vi "Configure Spurious Emission (Limit Setup).vi"(0 "VISA resource name":refnum<visa-resource-name>, 1 "Spurious Threshold":dbl[](array[numeric]) min=-200.0 max=50.0 format="%.2f", 2 "Spurious Stop Level Mode":i32[](array[ring]) items=["Auto", "Manual"], 5 "Spurious Absolute Level Start":dbl[](array[numeric]) min=-200.0 max=50.0 format="%.2f", 7 "Spurious Absolute Level Stop":dbl[](array[numeric]) min=-200.0 max=50.0 format="%.2f", 9 "Spurious Resolution":dbl[](array[numeric]) min=0.001 max=50.0 format="%.3f", 11 "error in (no error)":errorcluster) -> (4 "VISA resource name out":refnum<visa-resource-name>, 15 "error out":errorcluster)   [LabVIEW 2020, in "Anritsu Signal Analyzer Series.lvlib"]
doc: "Configures the Limit for Spurious Emission measurement."
uses:
  Anritsu Signal Analyzer Series.lvlib
panel:
  # "dBm"
  # "dBm"
  # "dBm"
  # "dB"
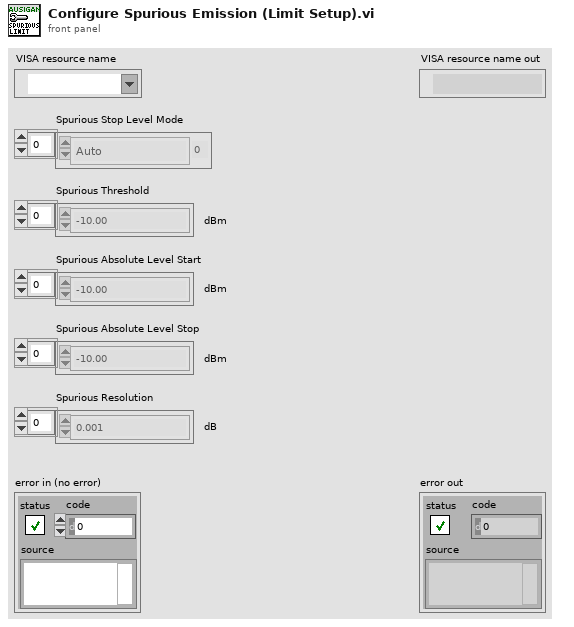
[diagram p1: front panel]
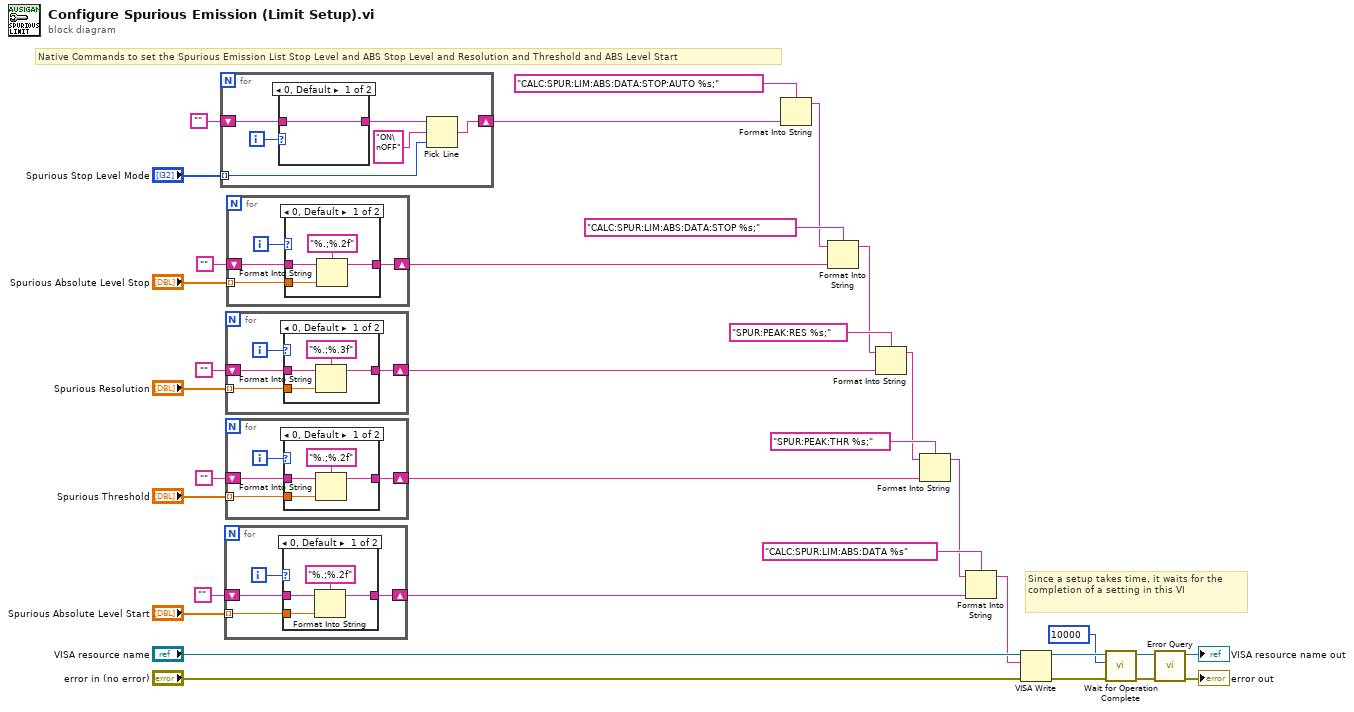
[diagram p0: block diagram]
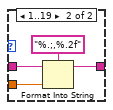
[diagram p2: hidden frame]
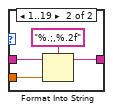
[diagram p3: hidden frame]
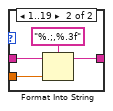
[diagram p4: hidden frame]
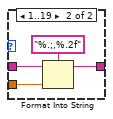
[diagram p5: hidden frame]
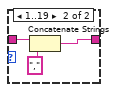
[diagram p6: hidden frame]
diagram:
  # "Since a setup takes time, it waits for the completion of a setting in this VI"
  # "Native Commands to set the Spurious Emission List Stop Level and ABS Stop Level and Resolution and Threshold and ABS Level Start"
  n1 = for {
    shift-right: [w35] -> w24
    shift-left: "" -> [w39]
    tunnel: "Spurious Stop Level Mode" -> [w36] mode=indexing
    i -> [w40]
    n2 = case shown="0, Default" w40 {
      tunnel: w39 -> [w41 w44]
      tunnel: [w41 w42] -> w37
      frame 0, Default {
      }
      frame 1..19 {
        n3 = Concatenate Strings(w44, "," ("string")) -> (w42:string)
      }
    }
    n4 = Pick Line(string ("")=w37, multi-line string="ON\nOFF" ("複数行文字列"), line index=w36) -> (output string=w35:string)
  }
  n5 = for {
    shift-right: [w45] -> w6
    shift-left: "" -> [w47]
    tunnel: "Spurious Absolute Level Start" -> [w46] mode=indexing
    i -> [w48]
    n6 = case shown="0, Default" w48 {
      tunnel: w47 -> [w51 w54]
      tunnel: [w49 w53] -> w45
      tunnel: w46 -> [w50 w55]
      frame 0, Default {
        n7 = Format Into String(format string="%.;%.2f" ("string"), initial string=w51, w50) -> (resulting string=w49:string)  [unwired: 1 in, 1 out]
      }
      frame 1..19 {
        n8 = Format Into String(format string="%.;,%.2f" ("string"), initial string=w54, w55) -> (resulting string=w53:string)  [unwired: 1 in, 1 out]
      }
    }
  }
  n9 = for {
    shift-right: [w57] -> w10
    shift-left: "" -> [w59]
    tunnel: "Spurious Resolution" -> [w58] mode=indexing
    i -> [w60]
    n10 = case shown="0, Default" w60 {
      tunnel: w59 -> [w63 w66]
      tunnel: [w61 w65] -> w57
      tunnel: w58 -> [w62 w67]
      frame 0, Default {
        n11 = Format Into String(format string="%.;%.3f" ("string"), initial string=w63, w62) -> (resulting string=w61:string)  [unwired: 1 in, 1 out]
      }
      frame 1..19 {
        n12 = Format Into String(format string="%.;,%.3f" ("string"), initial string=w66, w67) -> (resulting string=w65:string)  [unwired: 1 in, 1 out]
      }
    }
  }
  n13 = for {
    shift-right: [w69] -> w8
    shift-left: "" -> [w71]
    tunnel: "Spurious Threshold" -> [w70] mode=indexing
    i -> [w72]
    n14 = case shown="0, Default" w72 {
      tunnel: w71 -> [w75 w78]
      tunnel: [w73 w77] -> w69
      tunnel: w70 -> [w74 w79]
      frame 0, Default {
        n15 = Format Into String(format string="%.;%.2f" ("string"), initial string=w75, w74) -> (resulting string=w73:string)  [unwired: 1 in, 1 out]
      }
      frame 1..19 {
        n16 = Format Into String(format string="%.;,%.2f" ("string"), initial string=w78, w79) -> (resulting string=w77:string)  [unwired: 1 in, 1 out]
      }
    }
  }
  n17 = for {
    shift-right: [w81] -> w13
    shift-left: "" -> [w83]
    tunnel: "Spurious Absolute Level Stop" -> [w82] mode=indexing
    i -> [w84]
    n18 = case shown="0, Default" w84 {
      tunnel: w83 -> [w87 w90]
      tunnel: [w85 w89] -> w81
      tunnel: w82 -> [w86 w91]
      frame 0, Default {
        n19 = Format Into String(format string="%.;%.2f" ("string"), initial string=w87, w86) -> (resulting string=w85:string)  [unwired: 1 in, 1 out]
      }
      frame 1..19 {
        n20 = Format Into String(format string="%.;,%.2f" ("string"), initial string=w90, w91) -> (resulting string=w89:string)  [unwired: 1 in, 1 out]
      }
    }
  }
  n21 = Format Into String(format string="CALC:SPUR:LIM:ABS:DATA:STOP:AUTO %s;" ("_CommandSet"), w24) -> (resulting string=w21:string)  [unwired: 2 in, 1 out]
  n22 = Format Into String(format string="CALC:SPUR:LIM:ABS:DATA:STOP %s;" ("_CommandSet"), initial string=w21, w13) -> (resulting string=w11:string)  [unwired: 1 in, 1 out]
  n23 = Format Into String(format string="SPUR:PEAK:RES %s;" ("_CommandSet"), initial string=w11, w10) -> (resulting string=w18:string)  [unwired: 1 in, 1 out]
  n24 = Format Into String(format string="SPUR:PEAK:THR %s;" ("_CommandSet"), initial string=w18, w8) -> (resulting string=w16:string)  [unwired: 1 in, 1 out]
  n25 = Format Into String(format string="CALC:SPUR:LIM:ABS:DATA %s" ("_CommandSet"), initial string=w16, w6) -> (resulting string=w15:string)  [unwired: 1 in, 1 out]
  n26 = VISA Write(VISA resource name="VISA resource name", write buffer=w15, error in (no error)="error in (no error)") -> (VISA resource name out=w3:refnum<visa-resource-name>, error out=w2:errorcluster)  [unwired: 1 out]
  n27 = call "Wait for Operation Complete.vi"("error in (no error)"=w2, "Maximum Time (10000mSec)"=10000, "VISA resource name"=w3) -> ("error out"=w4:errorcluster, "VISA resource name out"=w5:refnum<visa-resource-name>)  [unwired: 7 in]
  n28 = call "Error Query.vi"("error in (no error)"=w4, "VISA resource name"=w5) -> ("error out"=→"error out":errorcluster, "VISA resource name out"=→"VISA resource name out":refnum<visa-resource-name>)  [unwired: 6 in, 2 out]
